vi "fftGetMags_IV.vi"(0 "input cluster":cluster{"f0":dbl, "df":dbl, "magnitude":dbl[]}, 5 "405 F (Hz)":i32, 7 "532 F (Hz)":i32, 9 "660 F (Hz)":i32, 11 "785 F (Hz)":i32, 12 "unit cal, scu":dbl=1000.0) -> (4 "mag405 (mV)":dbl, 6 "mag532 (mV)":dbl, 8 "mag660 (mV)":dbl, 10 "mag785 (mV)":dbl)   [LabVIEW 2011]
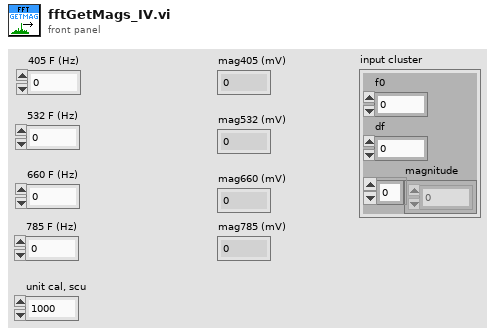
[diagram p1: front panel]
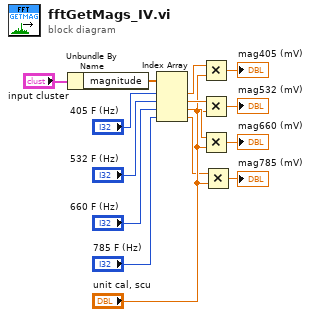
[diagram p0: block diagram]
diagram:
  n1 = Unbundle By Name("input cluster") -> ("magnitude"=w7:dbl[])
  n2 = Index Array(array=w7, index #1="405 F (Hz)", index #2="532 F (Hz)", index #3="660 F (Hz)", index #4="785 F (Hz)") -> (element #1=w10:dbl, element #2=w8:dbl, element #3=w9:dbl, element #4=w1:dbl)
  n3 = Multiply(x=w10, y="unit cal, scu") -> (x*y=→"mag405 (mV)":dbl)
  n4 = Multiply(x=w8, y="unit cal, scu") -> (x*y=→"mag532 (mV)":dbl)
  n5 = Multiply(x=w9, y="unit cal, scu") -> (x*y=→"mag660 (mV)":dbl)
  n6 = Multiply(x=w1, y="unit cal, scu") -> (x*y=→"mag785 (mV)":dbl)
